vi "离线AD原码转换成物理值 .vi"(7 "原始码":u16[](array[numeric]), 8 "错误输入":errorcluster caption="输出簇", 9 "AD数据个数":i32, 11 "文件句柄":i32) -> (0 "错误输出":errorcluster, 2 "AD物理值":dbl[](array[numeric]), 3 "文件句柄出":i32)   [LabVIEW 2011]
uses:
  dll/em9636.dll
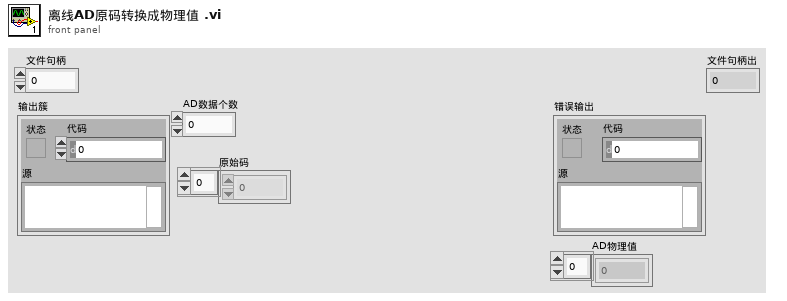
[diagram p1: front panel]
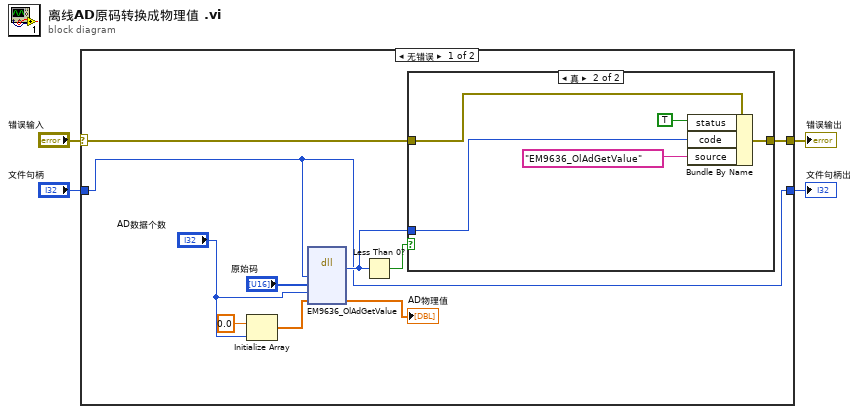
[diagram p0: block diagram]
diagram:
  n1 = case shown="无错误" "错误输入" {
    selector: "错误输入" -> [w10 w22]
    tunnel: [w12 w22] -> w3
    tunnel: "文件句柄" -> [w11 w21]
    tunnel: [w11 w21] -> w1
    frame No Error {
      n2 = Initialize Array(0.0 ("元素"), "AD数据个数") -> (w5:dbl[])
      n3 = dll-call lib="PTH1abs Eèµ éç LABVIEWæºVI(v2.0)EM9636BD)EM9636BDè°ç¨APIå½æ°æ¹æ³éè®¯ä¾ç¨EM9636_demo_labview2011dll\nem9636.dll" fn="EM9636_OlAdGetValue"("文件句柄"=w11, "AD原始码"="原始码", "AD原码个数"="AD数据个数", "AD物理值"=w5) -> ("错误信息"=w13:i32, "AD物理值"=→"AD物理值":dbl[])  [unwired: 6 in, 2 out]
      n4 = Less Than 0?(x=w13) -> (x < 0?=w14:bool)
      n5 = case shown="真" w14 {
        tunnel: [w15 w18] -> w12
        tunnel: w10 -> [w15 w20]
        tunnel: w13 -> [_ w17]
        frame False {
        }
        frame True {
          n6 = Bundle By Name(cluster=w20, "status"=TRUE, "code"=w17, "source"="EM9636_OlAdGetValue") -> (w18:errorcluster)
        }
      }
    }
    frame Error {
    }
  }
  "文件句柄出" <- w1
  "错误输出" <- w3
